vi "@Untitled #6.vi"() -> ()   [LabVIEW 2015]
uses:
  Controls/Sample Line State Enumerator.ctl
panel:
  out "x-y":i32(graph)
  out "data out":T1
  in  "Boolean":bool
  out "Interlock":bool
  # "02/06/15 08:18:22 AM @Sample Line: Error code -1950678963; \nSource:Read Variable in Interlock.lvclass:Read.vi:180001->\nInterlock Allow.lvclass:Read.vi:180001->\nInterlock.lvclass:Query Chain.vi:460002->\nSample Line.lvclass:Open Line.vi->\nOpen Line Msg.lvclass:Do.vi:3750001->\nActor Framework.lvlib:Actor.lvclass:Receive Message.vi:1040003->\nActor Framework.lvlib:Actor.lvclass:Actor Core.vi:5880003->\nCO2 Actor.lvclass:Actor Core.vi:5880001->Sample Line.lvclass:Actor Core.vi:5880001->\nActor Framework.lvlib:Actor.lvclass:Actor.vi:6640004->\nActor Framework.lvlib:Actor.lvclass:Actor.vi.ACBRProxyCaller.BF000001;\nError -1950678963 occurred at Read Variable in Interlock.lvclass:Read.vi:180001->\nInterlock Allow.lvclass:Read.vi:180001->Interlock.lvclass:Query Chain.vi:460002->\nSample Line.lvclass:Open Line.vi->Open Line Msg.lvclass:Do.vi:3750001->\nActor Framework.lvlib:Actor.lvclass:Receive Message.vi:1040003->\nActor Framework.lvlib:Actor.lvclass:Actor Core.vi:5880003->\nCO2 Actor.lvclass:Actor Core.vi:5880001->Sample Line.lvclass:Actor Core.vi:5880001->\nActor Framework.lvlib:Actor.lvclass:Actor.vi:6640004->\nActor Framework.lvlib:Actor.lvclass:Actor.vi.ACBRProxyCaller.BF000001\n\nPossible reason(s):\n\nLabVIEW:  Unable to open the variable connection. \nA connection to the specified variable is already open using a different data type."
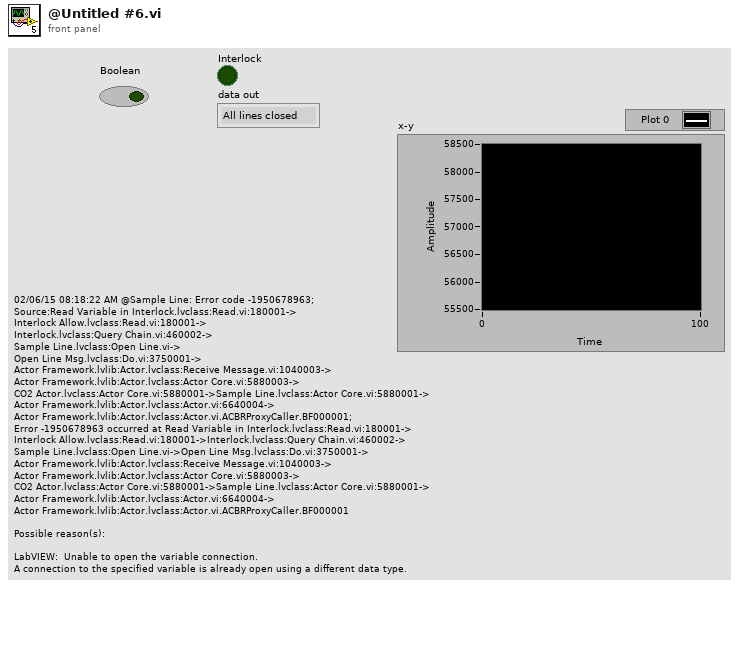
[diagram p1: front panel]
types:
  T1 = typedef "Sample Line State Enumerator.ctl" = enum16{"All lines closed", "Sample line 1.", "Sample line 2.", "Sample line 3.", "Sample line 4.", "Sample line 5.", "Out of range"}
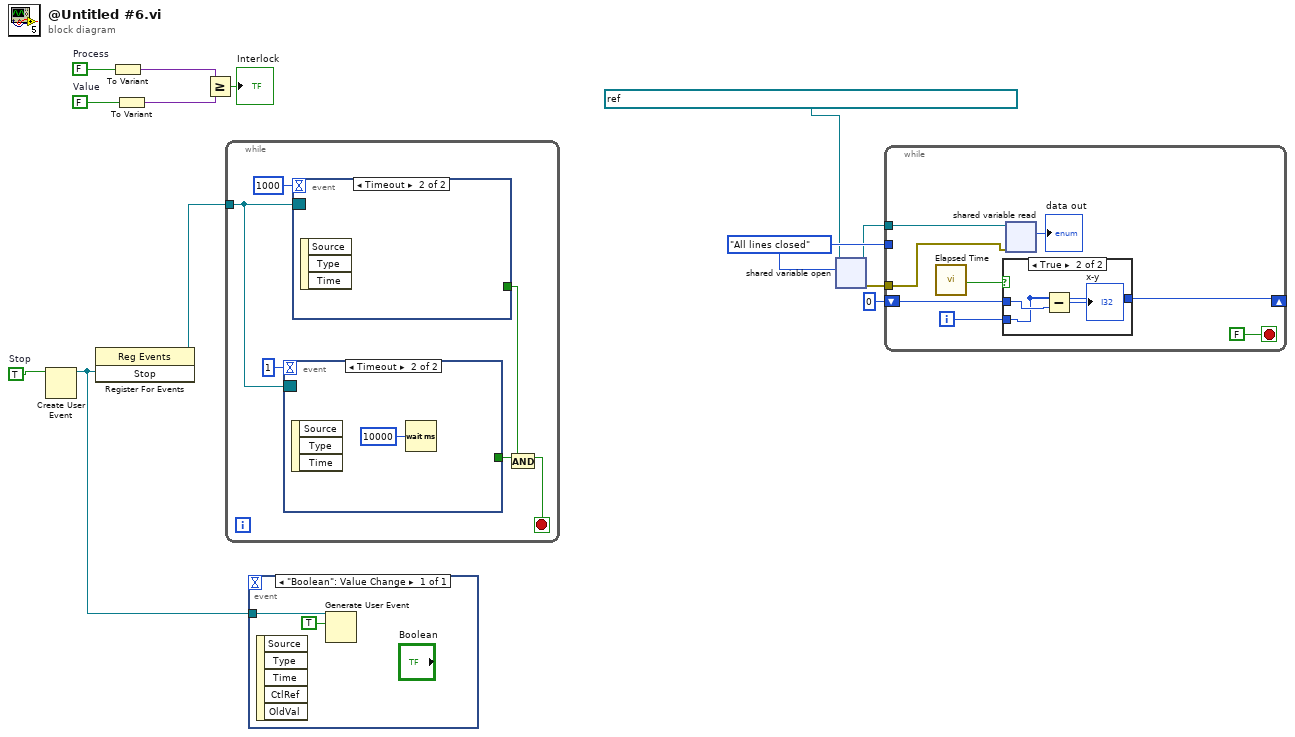
[diagram p0: block diagram]
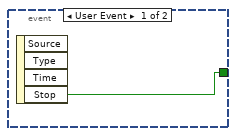
[diagram p3: hidden frame]
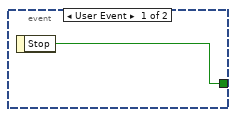
[diagram p4: hidden frame]
diagram:
  w3 = Sample_Line_State_Enumerator."All lines closed" ("Enum")
  w8 = TRUE  # Stop
  w13 = FALSE  # Process
  w12 = FALSE  # Value
  n1 = Create User Event(user event datatype=w8) -> (user event=w6:refnum<user-event>)  [unwired: 1 in, 1 out]
  n2 = register-events(w6) -> (reference out=w7:refnum<event-registration>)  [unwired: 2 in, 1 out]
  n3 = To Variant(anything=w13) -> (Variant=w10:variant)
  n4 = To Variant(anything=w12) -> (Variant=w9:variant)
  n5 = Greater Or Equal?(x=w10, y=w9) -> (x >= y?=→"Interlock":bool)
  n6 = while {
    tunnel: w7 -> [w19]
    stop <- w15 stop-if-true
    n7 = event shown="[1] Timeout" {
      selector: w19 -> [_ _]
      dyn-events: _ -> [_ _]
      timeout: 1 -> [_ _]
      tunnel: [w20 _] -> w16
      event User Event {
        n8 = event-data() -> ("Stop"=w20:bool)  [unwired: 1 in, 3 out]
      }
      event Timeout {
        n9 = event-data() -> ()  [unwired: 1 in, 3 out]
        n10 = Wait (ms)(milliseconds to wait=u32 10000) -> ()  [unwired: 1 out]
      }
    }
    n11 = event shown="[1] Timeout" {
      selector: w19 -> [_ _]
      dyn-events: _ -> [_ _]
      timeout: 1000 -> [_ _]
      tunnel: [w22 _] -> w14
      event User Event {
        n12 = event-data() -> ("Stop"=w22:bool)  [unwired: 1 in]
      }
      event Timeout {
        n13 = event-data() -> ()  [unwired: 1 in, 3 out]
      }
    }
    n14 = And(x=w16, y=w14) -> (x .and. y?=w15:bool)
  }
  n15 = event shown="[0] \"Boolean\": Value Change" {
    selector: _ -> [_]
    dyn-events: _ -> [_]
    timeout: _ -> [_]
    tunnel: w6 -> [w24]
    event "Boolean": Value Change {
      n16 = event-data() -> ()  [unwired: 1 in, 5 out]
      n17 = Generate User Event(user event=w24, event data cluster=TRUE ("event data")) -> ()  [unwired: 2 in, 2 out]
    }
  }
  n18 = shared-variable-open(refnum<k21> "ni.var.psp://localhost/AMS Gas SHV PC/Sample Lines/Sample Line Status" ("shared variable refnum in"), w3) -> (w1:refnum<k21>, w4:errorcluster)  [unwired: 2 in]
  n19 = while {
    shift-right: [w27] -> _
    shift-left: 0 -> [w29]
    tunnel: w3 -> [_]
    tunnel: w4 -> [w25]
    tunnel: w1 -> [w32]
    i -> [w28]
    stop <- FALSE stop-if-true
    n20 = call "Elapsed Time"() -> ("Time has Elapsed"=w30:bool)  [unwired: 12 in, 7 out]
    n21 = case shown="True" w30 {
      tunnel: w29 -> [w33 w36]
      tunnel: w28 -> [_ w34]
      tunnel: [w33 w34] -> w27
      frame False {
      }
      frame True {
        n22 = Subtract(x=w34, y=w36) -> (x-y=→"x-y":i32)
      }
    }
    n23 = shared-variable-read(w32, w25) -> (→"data out":T1)  [unwired: 3 out]
  }
